vi "colorDist.vi"(5 "Reference Colour":u32(colorbox), 6 "error in":errorcluster, 7 "B":dbl, 8 "G":dbl, 9 "R":dbl) -> (0 "error out":errorcluster, 2 "intensity":dbl, 3 "delta":dbl)   [LabVIEW 2013]
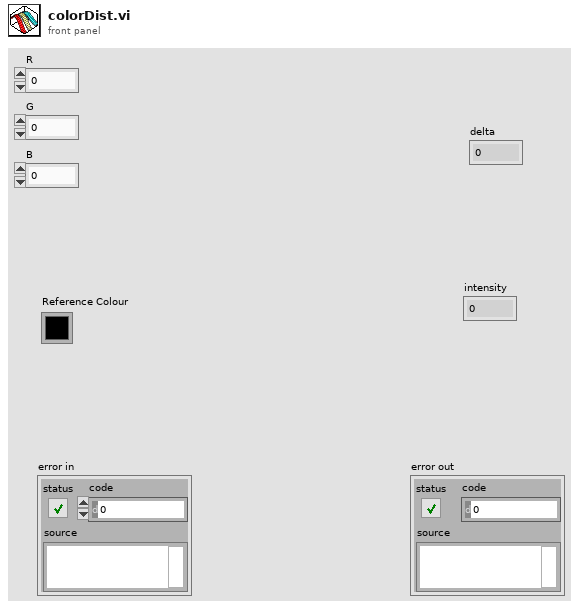
[diagram p1: front panel]
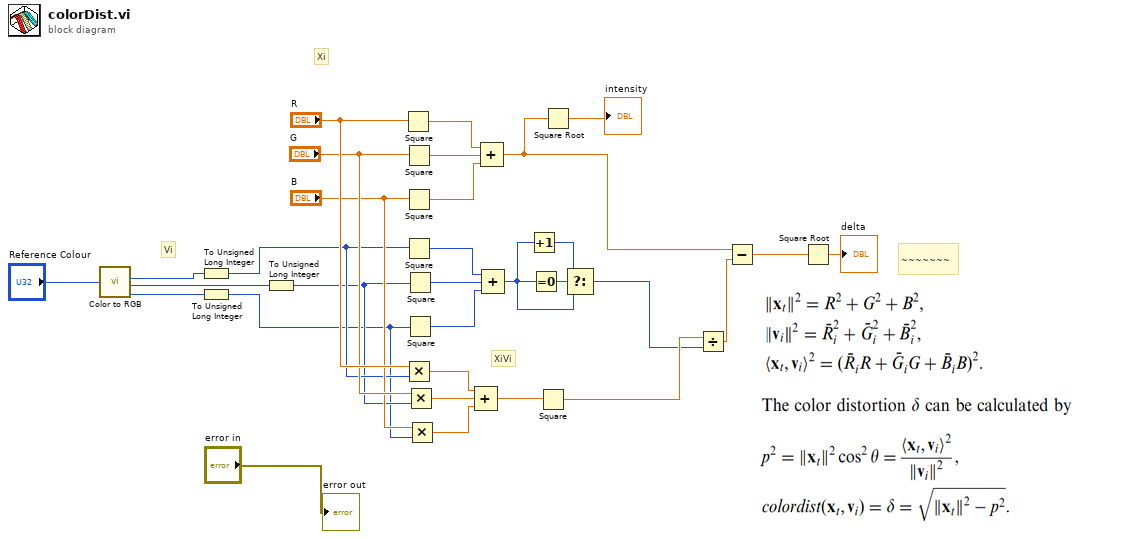
[diagram p0: block diagram]
diagram:
  # "XiVi"
  # "Vi"
  # "Xi"
  # "~~~~~~~"
  n1 = call <vilib>:"Color to RGB.vi"("Color"="Reference Colour") -> ("R"=w6:u8, "G"=w7:u8, "B"=w4:u8)  [unwired: 1 out]
  n2 = To Unsigned Long Integer(number=w6) -> (unsigned 32bit integer=w8:u32)
  n3 = To Unsigned Long Integer(number=w4) -> (unsigned 32bit integer=w3:u32)
  n4 = To Unsigned Long Integer(number=w7) -> (unsigned 32bit integer=w5:u32)
  n5 = Square(x="R") -> (x^2=w21:dbl)
  n6 = Square(x="G") -> (x^2=w22:dbl)
  n7 = Square(x="B") -> (x^2=w23:dbl)
  n8 = Square(x=w8) -> (x^2=w24:u32)
  n9 = Multiply(x="R", y=w8) -> (x*y=w27:dbl)
  n10 = Square(x=w5) -> (x^2=w25:u32)
  n11 = Square(x=w3) -> (x^2=w26:u32)
  n12 = Multiply(x="G", y=w5) -> (x*y=w28:dbl)
  n13 = Multiply(x="B", y=w3) -> (x*y=w29:dbl)
  n14 = Compound Arithmetic op=ADD(w27, w28, w29) -> (w13:dbl)
  n15 = Compound Arithmetic op=ADD(w21, w22, w23) -> (w2:dbl)
  n16 = Compound Arithmetic op=ADD(w24, w25, w26) -> (w9:u32)
  n17 = Increment(x=w9) -> (x+1=w10:u32)
  n18 = Equal To 0?(x=w9) -> (x = 0?=w11:bool)
  n19 = Square(x=w13) -> (x^2=w12:dbl)
  n20 = Square Root(x=w2) -> (sqrt(x)=→"intensity":dbl)
  n21 = Select(t=w10, s=w11, f=w9) -> (s? t:f=w1:u32)
  n22 = Divide(x=w12, y=w1) -> (x/y=w30:dbl)
  n23 = Subtract(x=w2, y=w30) -> (x-y=w31:dbl)
  n24 = Square Root(x=w31) -> (sqrt(x)=→"delta":dbl)
  "error out" <- "error in"
